vi "Add Text Node with Attributes.vi"(4 "Attr Value":string="CodeDocumentation", 6 "Attr Name":string="CodeDocumentation", 7 "Tag Name":string="CodeDocumentation", 8 "error in":errorcluster, 9 "Tag Data":string, 10 "Element in":refnum<k20>, 11 "Document in":refnum<k20>) -> (0 "error out":errorcluster, 2 "Element out":refnum<k20>, 3 "Document out":refnum<k20>)   [LabVIEW 2026]
uses:
  <resource>/objmgr/DOMUserDefRef.rc
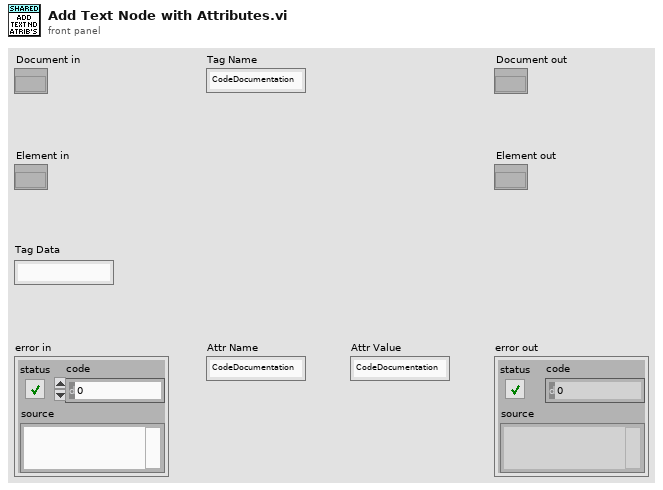
[diagram p1: front panel]
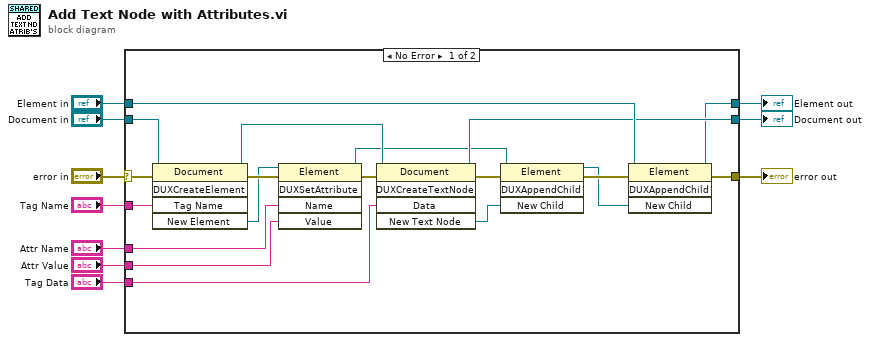
[diagram p0: block diagram]
diagram:
  n1 = case shown="No Error" "error in" {
    selector: "error in" -> [w20 w30]
    tunnel: "Tag Name" -> [w28 _]
    tunnel: "Tag Data" -> [w19 _]
    tunnel: "Document in" -> [w25 w31]
    tunnel: "Element in" -> [w24 w32]
    tunnel: [w23 w31] -> w6
    tunnel: [w22 w32] -> w5
    tunnel: [w21 w30] -> w4
    tunnel: "Attr Name" -> [w12 _]
    tunnel: "Attr Value" -> [w11 _]
    frame No Error {
      n2 = invoke class="Document" method="DUXCreateElement"(reference=w25, error in=w20, "Tag Name"=w28) -> (reference out=w27:refnum<k20>, error out=w16:errorcluster, "New Element"=w14:refnum<k20>)  [unwired: 2 in, 2 out]
      n3 = invoke class="Element" method="DUXSetAttribute"(reference=w14, error in=w16, "Name"=w12, "Value"=w11) -> (reference out=w13:refnum<k20>, error out=w15:errorcluster)  [unwired: 1 in, 3 out]
      n4 = invoke class="Document" method="DUXCreateTextNode"(reference=w27, error in=w15, "Data"=w19) -> (reference out=w23:refnum<k20>, error out=w17:errorcluster, "New Text Node"=w18:refnum<k20>)  [unwired: 2 in, 2 out]
      n5 = invoke class="Element" method="DUXAppendChild"(reference=w13, error in=w17, "New Child"=w18) -> (reference out=w26:refnum<k20>, error out=w29:errorcluster)  [unwired: 1 in, 2 out]
      n6 = invoke class="Element" method="DUXAppendChild"(reference=w24, error in=w29, "New Child"=w26) -> (reference out=w22:refnum<k20>, error out=w21:errorcluster)  [unwired: 1 in, 2 out]
    }
    frame Error {
    }
  }
  "error out" <- w4
  "Document out" <- w6
  "Element out" <- w5
